vi "DHE_SetTimingInfo.vi"(10 "Timing":T2={"PixelTime"=1.0, "SkipPixel"=1.0, "SkipRow"=1.0, "ShiftRow"=1.0, "ShiftedPix"=1, "known_overhead"=1.0, "DET_READ_TIME"=1.0} {"DET_READ_TIME" format="%.2f"; "known_overhead" format="%.2f"; "ShiftRow" format="%.2f"; "SkipRow" format="%.2f"; "SkipPixel" format="%.2f"; "PixelTime" format="%.2f"}, 11 "Database RefNum out":T1) -> ()   [LabVIEW 2016]
uses:
  Common/public/vis/CMN_TimingInfo.ctl
  DBSHAND/private/vis/DatabaseHand_RefNum.ctl
  private/vis/DHE_GBLDriverVariables.vi
  DBSHAND/private/vis/DatabaseHand_Element_Set(single).vi
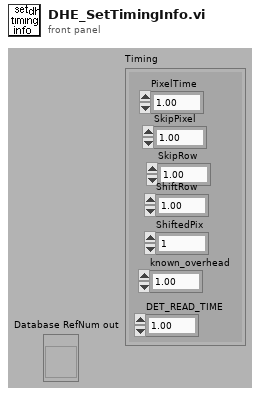
[diagram p1: front panel]
types:
  T1 = typedef "DatabaseHand_RefNum.ctl" = refnum<vi>
  T2 = typedef "CMN_TimingInfo.ctl" = cluster{"PixelTime":sgl, "SkipPixel":sgl, "SkipRow":sgl, "ShiftRow":sgl, "ShiftedPix":u16, "known_overhead":sgl, "DET_READ_TIME":sgl}
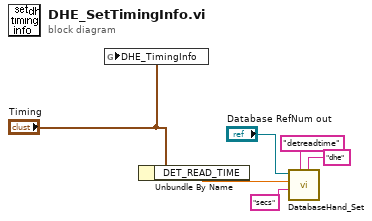
[diagram p0: block diagram]
diagram:
  n1 = global write "DHE_GBLDriverVariables.vi" "DHE_TimingInfo"("Timing") -> ()
  n2 = Unbundle By Name("Timing") -> ("DET_READ_TIME"=w5:sgl)
  n3 = call-poly "DatabaseHand_Set.vi"("group"="dhe", "name"="detreadtime", "unit"="secs", "value"=w5, "Database RefNum in"="Database RefNum out") -> ()  [unwired: 3 in, 4 out]
